vi "OpenImaqSession.vi"(8 "error in (no error)":errorcluster, 10 "camera settings":T2, 11 "interface name":string) -> (0 "error out":errorcluster, 3 "imaq session":T1)   [LabVIEW 2017, in "IrAcquisition.lvlib"]
uses:
  <vilib>/addons/InsightCM/Devices/Shared/Ir/IrAcquisition/IrAcquisition.lvlib
  <vilib>/addons/InsightCM/Devices/Shared/Ir/IrAcquisition/controls/IRCameraSettings.ctl
  <vilib>/userdefined/High Color/IMAQdx.ctl
  <vilib>/vision/driver/NI_Vision_Acquisition_Software.lvlib
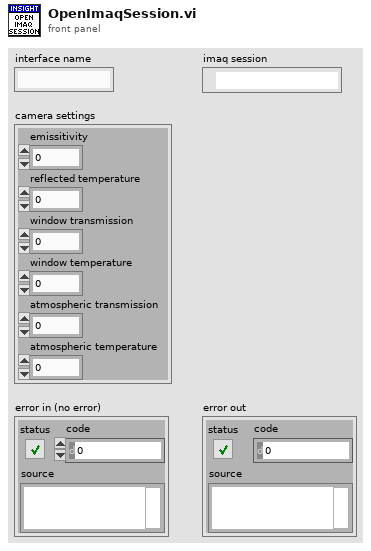
[diagram p1: front panel]
types:
  T1 = typedef "IMAQdx.ctl" = refnum<k21>
  T2 = typedef "IrAcquisition.lvlib/IRCameraSettings.ctl" = cluster{"emissitivity":dbl, "reflected temperature":dbl, "window transmission":dbl, "window temperature":dbl, "atmospheric transmission":dbl, "atmospheric temperature":dbl}
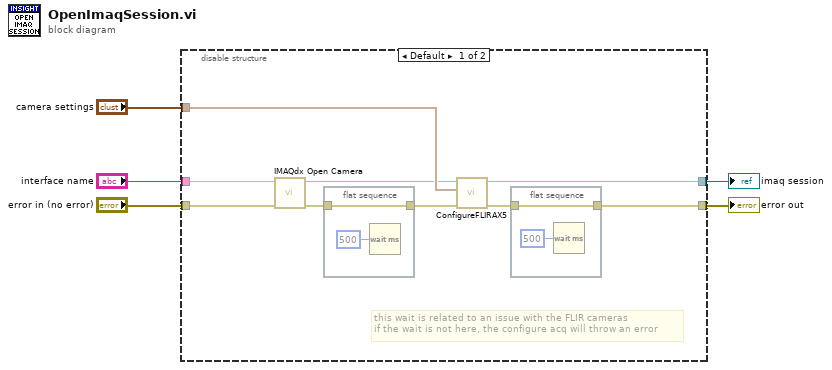
[diagram p0: block diagram]
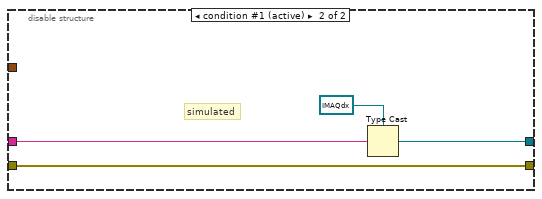
[diagram p2: hidden frame]
diagram:
  n1 = disable-structure shown="Default" {
    disable-tunnel: "error in (no error)" -> [w14 w22]
    disable-tunnel: [w13 w22] -> w4
    disable-tunnel: "camera settings" -> [w12 _]
    disable-tunnel: [w8 w19] -> w2
    disable-tunnel: "interface name" -> [w6 w21]
    frame condition #0 {
      # "this wait is related to an issue with the FLIR cameras\nif the wait is not here, the configure acq will throw an error"
      n2 = call <vilib>:"IMAQdx Open Camera.vi"("error in"=w14, "Session In"=w6) -> ("error out"=w10:errorcluster, "Session Out"=w7:T1)  [unwired: 1 in, 7 out]
      n3 = flat-sequence {
        tunnel: w10 -> [w16]
        tunnel: [w16] -> w11
        frame #0 {
          n4 = Wait (ms)(milliseconds to wait=u32 500) -> ()  [unwired: 1 out]
        }
      }
      n5 = call <vilib>:"ConfigureFLIRAX5.vi"("error in (no error)"=w11, "IR camera settings"=w12, "IMAQdx Session"=w7) -> ("error out"=w9:errorcluster, "IMAQdx Session out"=w8:T1)  [unwired: 7 in]
      n6 = flat-sequence {
        tunnel: w9 -> [w18]
        tunnel: [w18] -> w13
        frame #0 {
          n7 = Wait (ms)(milliseconds to wait=u32 500) -> ()  [unwired: 1 out]
        }
      }
    }
    frame condition #1 (active) {
      # "simulated"
      n8 = Type Cast(type=T1 refnum ("imaq session"), x=w21) -> (*(type *) &x=w19:T1)
    }
  }
  "error out" <- w4
  "imaq session" <- w2
